vi "Get Value by Array (Object).vi"(8 "error in (no error)":errorcluster, 10 "Keys":string[](array[string]), 11 "JSON Object in":refnum<class "JSON Object.lvclass">) -> (0 "error out":errorcluster, 2 "JSON Object out":refnum<class "JSON Object.lvclass">)   [LabVIEW 2015, in "LVJSON.lvlib" / "JSON Object.lvclass"]
uses:
  JSON Object.lvclass
  JSON Helper/To More Specific Type (Object).vi
  JSON Helper/JSON Helper.lvclass
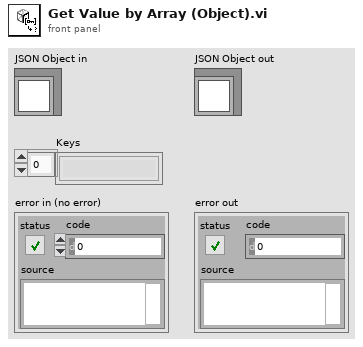
[diagram p1: front panel]
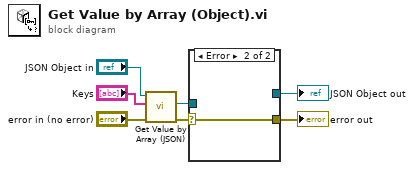
[diagram p0: block diagram]
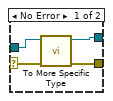
[diagram p2: hidden frame]
diagram:
  n1 = call "Get Value by Array (JSON).vi"("error in (no error)"="error in (no error)", "Keys"="Keys", "JSON Object in"="JSON Object in") -> ("error out"=w4:errorcluster, "JSON Datatype out"=w3:refnum<class "JSON Null.lvclass">)  [unwired: 7 in]
  n2 = case shown="Error" w4 {
    selector: w4 -> [w11 w12]
    tunnel: w3 -> [w10 _]
    tunnel: [w9 _] -> w2
    tunnel: [w8 w12] -> w1
    frame No Error {
      n3 = call-poly "To More Specific Type.vi"("error in (no error)"=w11, "JSON Datatype in"=w10) -> ("error out"=w8:errorcluster, "JSON Datatype out"=w9:refnum<class "JSON Object.lvclass">)  [unwired: 8 in]
    }
    frame Error {
    }
  }
  "JSON Object out" <- w2
  "error out" <- w1
